vi "PlotMieCurveFromRI.vi"(1 "Extinction ExtinctionUncertainity Size parameter and Number ofS sizes":T1, 2 "refractive index, imaginary":sgl step=0.01 format="%.3f", 3 "max size parameter alpha\n(alpha = 2Pi*r/lambda)":sgl=20.0 step=0.01 format="%.2f", 4 "refractive index, real":sgl=1.3 step=0.01 format="%.3f") -> (0 "Extinction Graph":cluster{"Ramp Pattern":dbl[], dbl[]}(graph))   [LabVIEW 2011]
uses:
  BaesDataTypeDefinition.ctl
  <vilib>/Analysis/1siggen.llb/Ramp Pattern by Samples.vi
  <vilib>/imath/engines/lvmath2/RunTimeEngine/NodeEndStatement/NIMS_NodeEndStatement_Output.vi
  <instcachedir>/0/NIMS_NodeEndStatement_Output_53EC0D466D134D7ABD903AC30B43404B.lvgen/NIMS_NodeEndStatement_Output_53EC0D466D134D7ABD903AC30B43404B_001.vi
  <vilib>/imath/engines/lvmath2/RunTimeEngine/ErrorHandling/NIMS_Finalize Error.vi
  mie2.dll
  <vilib>/Analysis/NI_AALBase.lvlib
panel:
  in  "Number of particle sizes for expected values":i32=1000
  out "totalscatter":sgl=2.73535
  out "backscatter":sgl=1.1527499
  out "<cos(theta)> 2":sgl=0.84980327
  out "extinction":sgl=2.7353504
  in  "angles (will compute\n2*angles-1 points from\n0...180 degrees)":u32=2
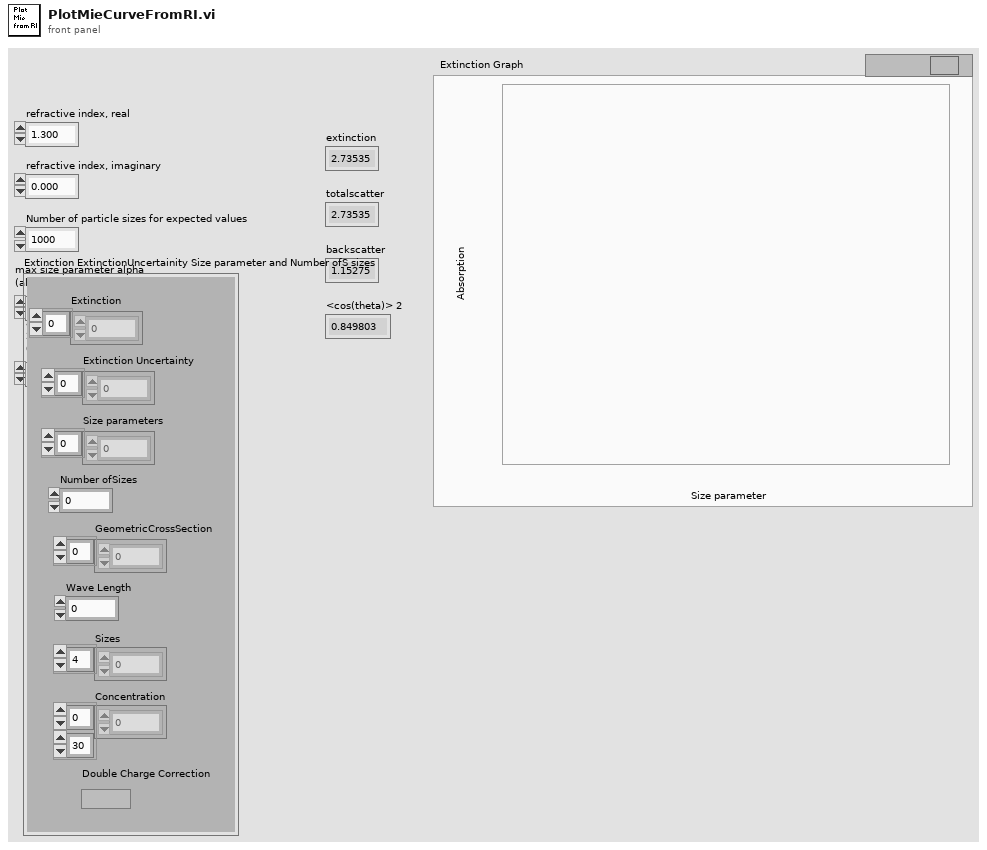
[diagram p1: front panel]
types:
  T1 = typedef "BaesDataTypeDefinition.ctl" = cluster{"Extinction":dbl[], "Extinction Uncertainty":dbl[], "Size parameters":dbl[], "Number ofSizes":dbl, "GeometricCrossSection":dbl[], "Wave Length":dbl, "Sizes":dbl[], "Concentration":dbl[][], "Double Charge Correction":bool}
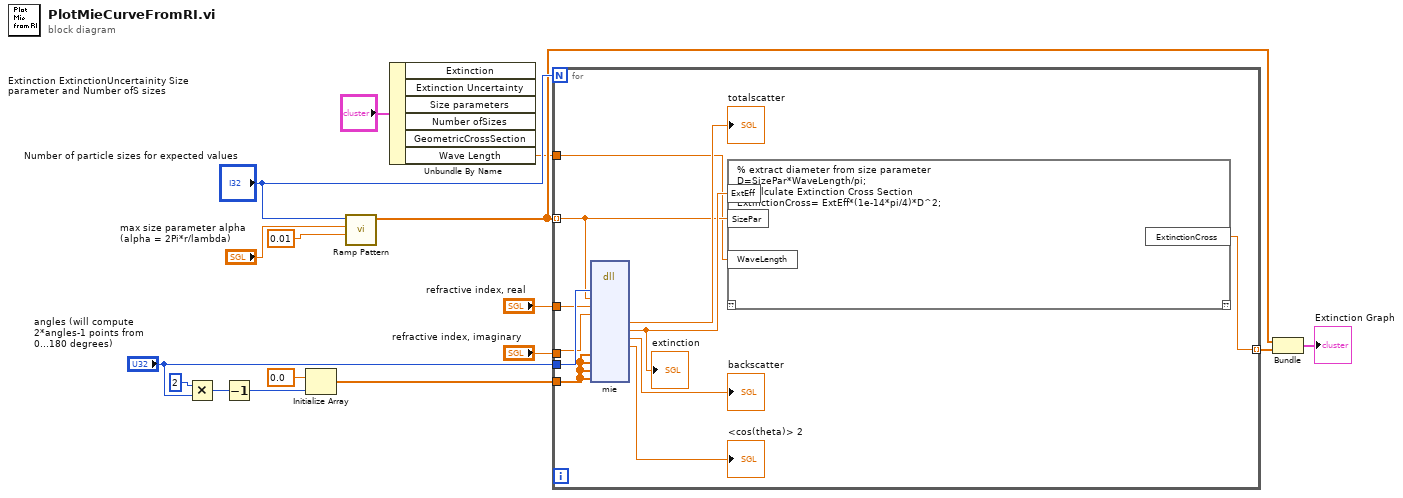
[diagram p0: block diagram]
diagram:
  n1 = Multiply(x=u32 2, y="angles (will compute\n2*angles-1 points from\n0...180 degrees)") -> (x*y=w15:u32)
  n2 = Decrement(x=w15) -> (x-1=w13:u32)
  n3 = Initialize Array(sgl 0.0, w13) -> (w7:sgl[])
  n4 = call-poly <vilib>:"Ramp Pattern.vi"("start"=0.01, "end"="max size parameter alpha\n(alpha = 2Pi*r/lambda)", "samples"="Number of particle sizes for expected values") -> ("Ramp Pattern"=w5:dbl[])  [unwired: 7 in, 1 out]
  n5 = Unbundle By Name("Extinction ExtinctionUncertainity Size parameter and Number ofS sizes") -> ("Wave Length"=w1:dbl)  [unwired: 5 out]
  n6 = for {
    N: "Number of particle sizes for expected values" -> [_]
    tunnel: w7 -> [w25]
    tunnel: "angles (will compute\n2*angles-1 points from\n0...180 degrees)" -> [w24]
    tunnel: "refractive index, real" -> [w23]
    tunnel: "refractive index, imaginary" -> [w22]
    tunnel: w5 -> [w19] mode=indexing
    tunnel: [w17] -> w4 mode=indexing
    tunnel: w1 -> [w18]
    n7 = dll-call lib="Z:/Dropbox/Lior Segev/Lior Segev Projects/RI retrieval in Labview/RIRetrievalInLabViewVer2/mie2.dll" fn="mie"("angles"=w24, "x"=w19, "r"=w23, "i"=w22, "spol_real"=w25, "spol_imaginary"=w25, "ppol_real"=w25, "ppol_imaginary"=w25) -> ("totalscatter"=→"totalscatter":sgl, "extinction"=w20:sgl, "backscatter"=→"backscatter":sgl, "<cos(theta)>"=→"<cos(theta)> 2":sgl)  [unwired: 16 in, 2 out]
    "extinction" <- w20
    n8 = mathscript code="% extract diameter from size parameter\nD=SizePar*WaveLength/pi;\n% Calculate Extinction Cross Section\nExtinctionCross= ExtEff*(1e-14*pi/4)*D^2;"("ExtEff"=w20, "SizePar"=w19, "WaveLength"=w18) -> ("ExtinctionCross"=w17:dbl)  [unwired: 1 in, 1 out]
  }
  n9 = Bundle("Ramp Pattern"=w5, w4) -> (→"Extinction Graph":cluster{"Ramp Pattern":dbl[], dbl[]})  [unwired: 1 in]
